vi "shooter_globals.vi"() -> ()   [LabVIEW 2020]
panel:
  in  "Flywheel Command":bool
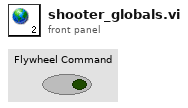
[diagram p1: front panel]
diagram:
